vi "aptControl.vi"() -> (0 "Moving":bool, 3 "Current Position":sgl)   [LabVIEW 2012]
uses:
  <vilib>/DAQmx/write.llb/DAQmx Write (Digital 1D Bool 1Chan 1Samp).vi
  <vilib>/DAQmx/write.llb/DAQmx Write (Analog Wfm 1Chan NSamp).vi
  <vilib>/DAQmx/read.llb/DAQmx Read (Analog Wfm 1Chan NSamp).vi
  <vilib>/DAQmx/miscellaneous.llb/DAQmx Fill In Error Info.vi
  <vilib>/Analysis/baseanly.llb/Mean (DBL).vi
  <vilib>/Utility/file.llb/Write To Spreadsheet File (DBL).vi
  <vilib>/Utility/file.llb/Read From Spreadsheet File (DBL).vi
  <vilib>/gmath/NI_Gmath.lvlib
  <vilib>/Analysis/NI_AALBase.lvlib
panel:
  out "Power Min&Max":i32[](array[numeric])
  out "Setup":i32
  out "MirrorPosition":sgl
  out "SavePath":path
  out "MinPos":sgl
  out "MaxPos":sgl
  out "Scaner":string
  in  "Tab Control":enum32{"Control", "Curve", "Calibrate"}(tab)
  in  "Shutter":bool
  in  "Power (mW)":dbl format="%#.0f"
  in  "Possition (0:360)":dbl format="%#.2f"
  in  "Up":bool
  in  "Down":bool
  in  "Mirror\nOverride":bool
  in  "Galvo":bool=TRUE caption="AOD"
  in  "Lens":u16(ring)=10 items=["4X"=4, "10X"=10, "16X"=16, "20X"=20, "25X"=25, "40X"=40, "60X"=60]
  out "Error/Wait":bool
  in  "Home":bool
  in  "stop":bool
  in  "Auto":bool
  out "Calibration Used":string
  out "Curve":cluster{"all rows":dbl[], "all rows":dbl[]}(graph)
  out "Curve 2":cluster{i32[], i32[]}(graph)
  in  "Path":path=path "X:/2Pcalibration"
  in  "Start Calibration":bool
  in  "WaveLengths":dbl[](array[numeric])=[800.0, 890.0]
  out "Finished":bool
  in  "quit":bool
  out "Remaining\n min":dbl format="%#.2f"
  out "Acquiring":bool
  out "Waiting":bool
  out "Moving 2":bool
  in  "Repetitions":dbl=1.0
  in  "Step Size":dbl=4.0
  out "Current mW":dbl format="%#.0f"
  out "Old possition":sgl
  in  "AOD motor":refnum<k7>(container)
  in  "Target Position":dbl
  in  "Attenuator motor":refnum<k7>(container)
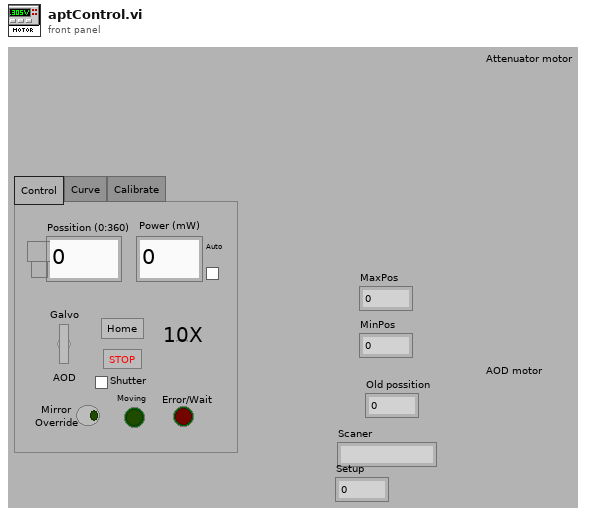
[diagram p1: front panel]
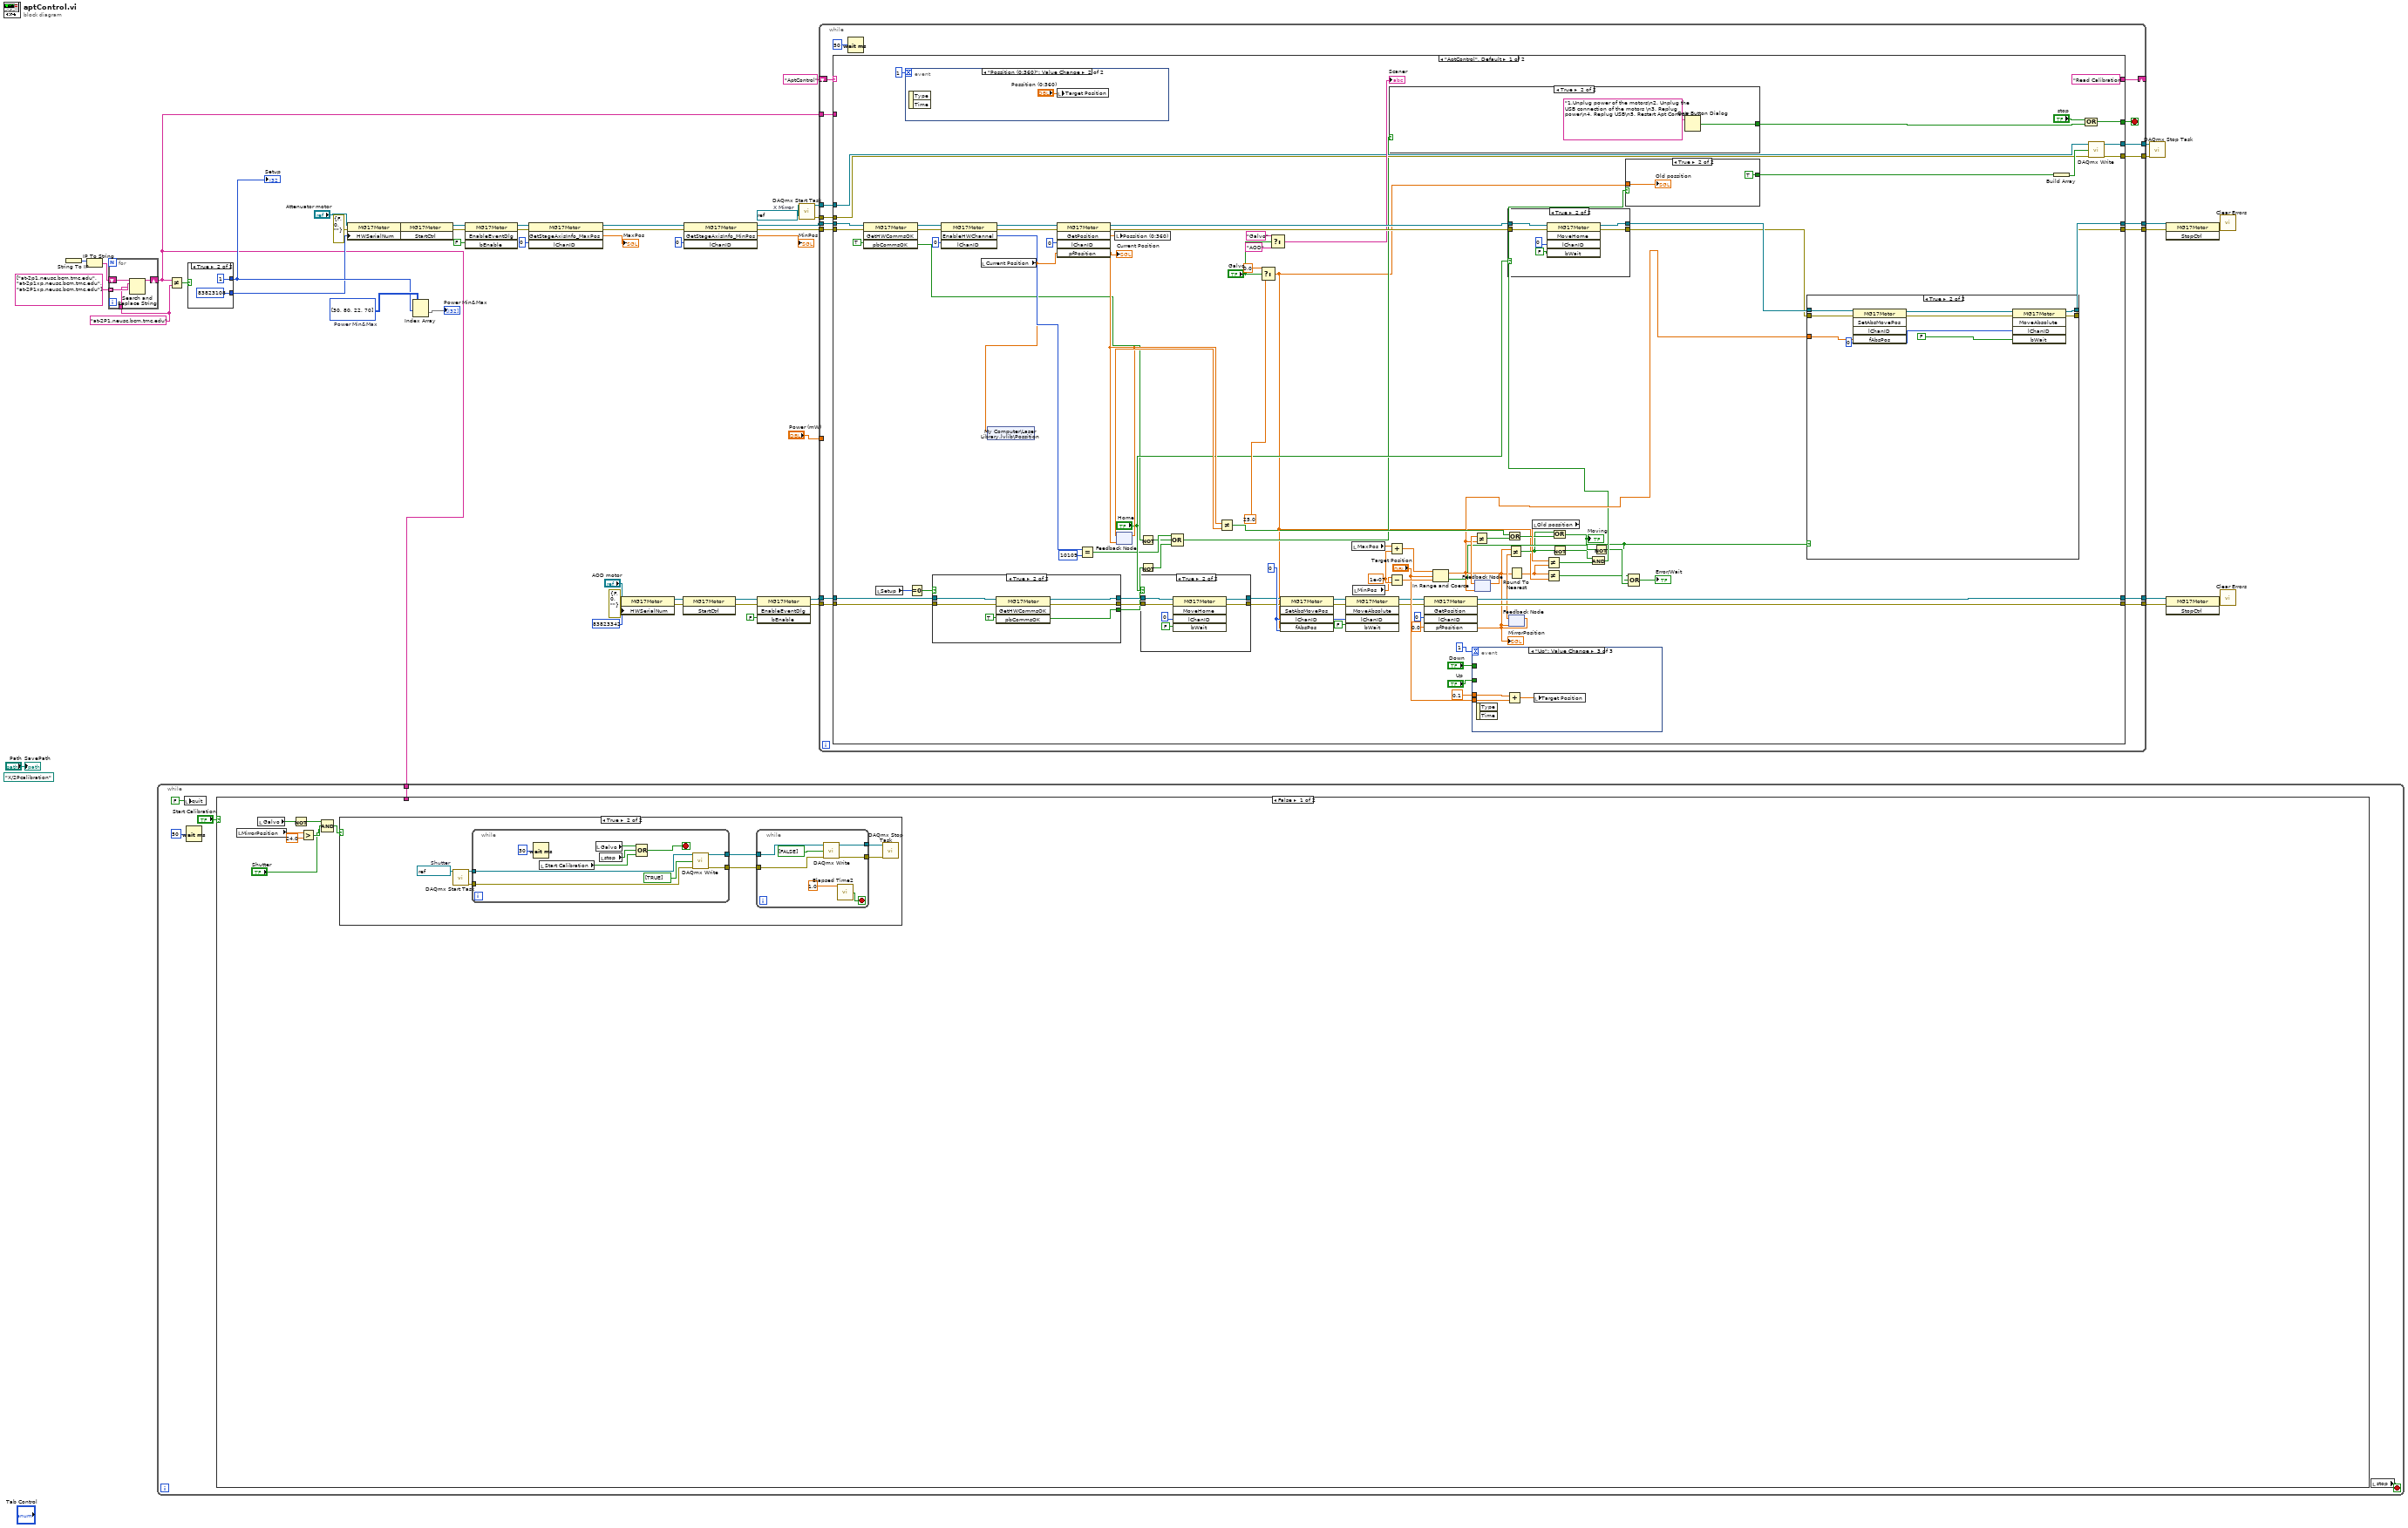
[diagram p0: block diagram]
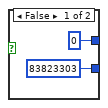
[diagram p2: hidden frame]
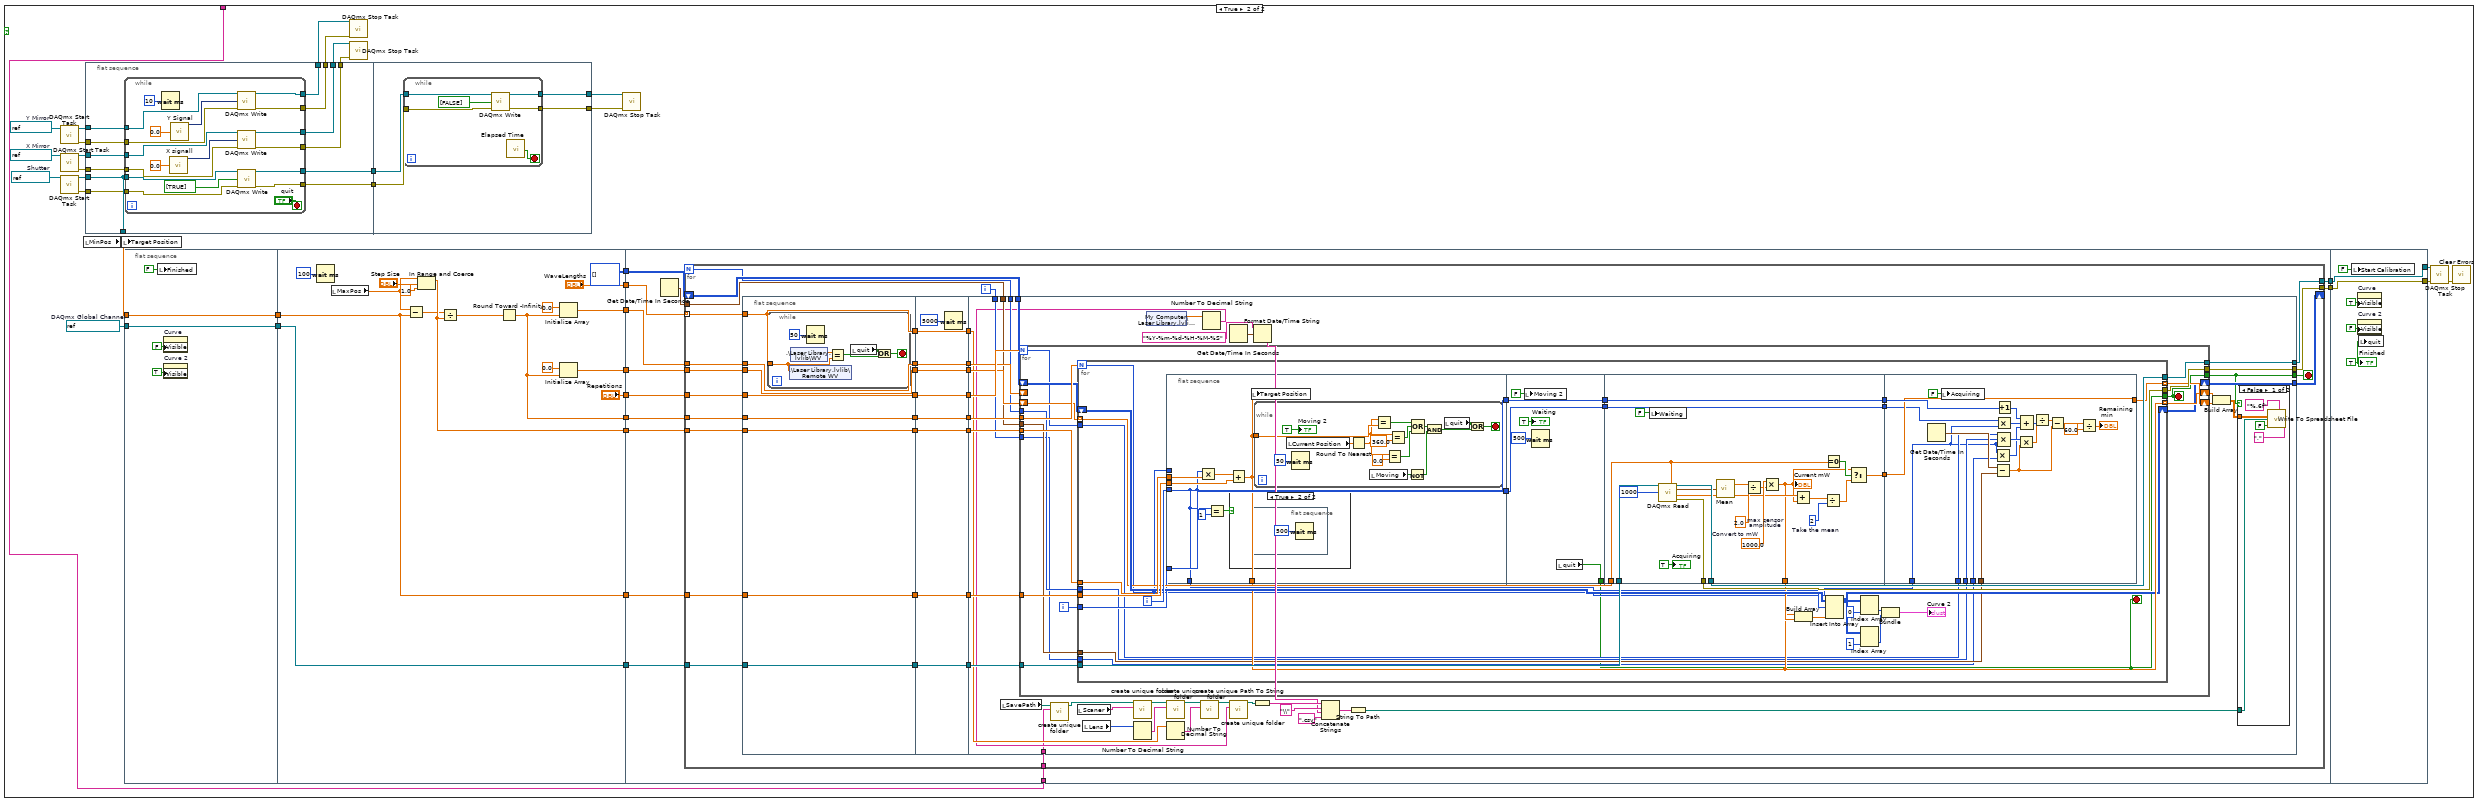
[diagram p4: hidden frame]
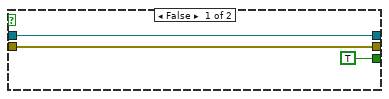
[diagram p7: hidden frame]
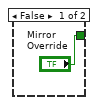
[diagram p9: hidden frame]
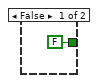
[diagram p10: hidden frame]
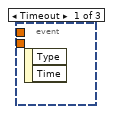
[diagram p11: hidden frame]
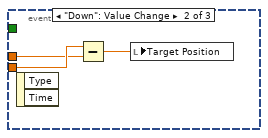
[diagram p12: hidden frame]
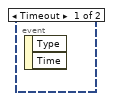
[diagram p13: hidden frame]
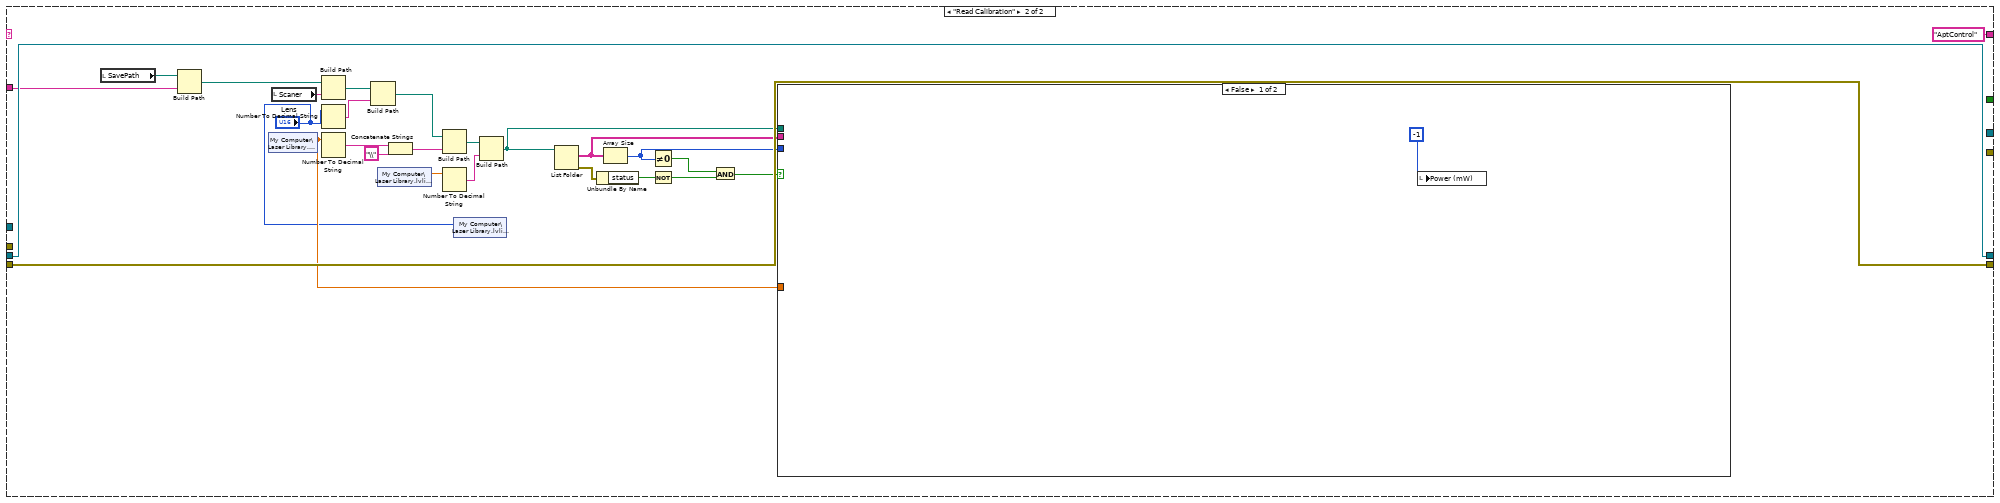
[diagram p16: hidden frame]
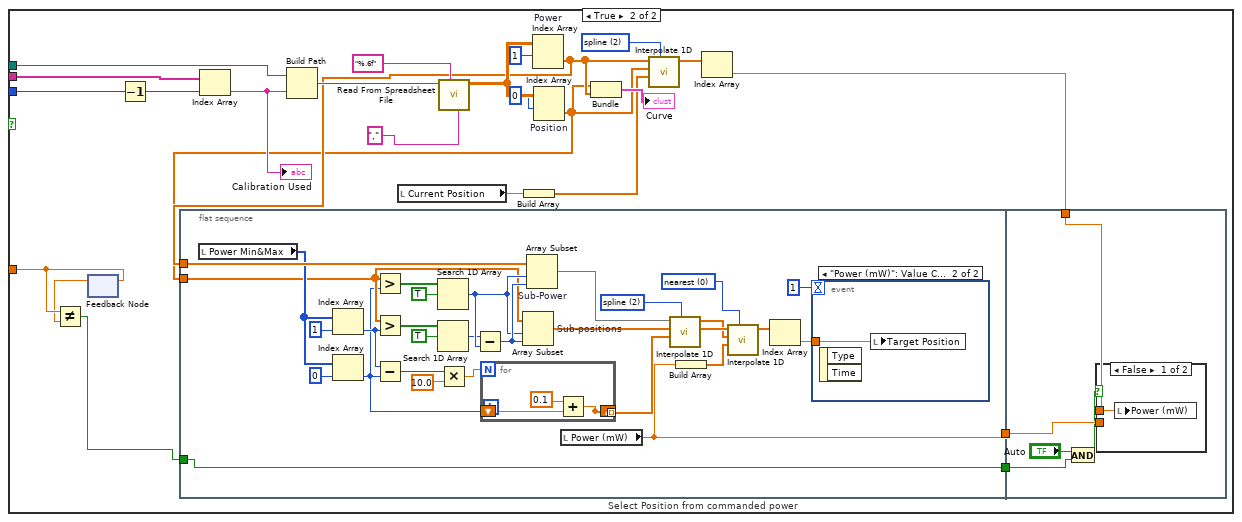
[diagram p17: hidden frame]
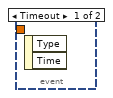
[diagram p18: hidden frame]
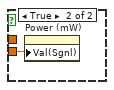
[diagram p19: hidden frame]
diagram:
  w2 = "at-2P1.neusc.bcm.tmc.edu"
  w11 = i32[][] [[30, 80], [22, 70]]  # Power Min&Max
  (unwired) path "X:/2Pcalibration"
  w20 = refnum<k21> "FlipMirror"  # X Mirror
  n1 = String To IP() -> (0:w8:u32)  [unwired: 1 in]
  n2 = IP To String(2:w8) -> (0:w3:string)  [unwired: 1 in]
  n3 = for {
    tunnel: string[] ["at-2p1.neusc.bcm.tmc.edu", "at-2p1xp.neusc.bcm.tmc.edu", "at-2P1xp.neusc.bcm.tmc.edu"] -> [w55] mode=indexing
    shift-right: [w53] -> w1
    shift-left: w3 -> [w54]
    tunnel: w2 -> [w52]
    n4 = Search and Replace String(input string=w54, search string=w55, replace string=w52) -> (result string=w53:string)  [unwired: 5 in, 3 out]
  }
  n5 = while {
    tunnel: w1 -> [w56]
    stop <- w59 stop-if-true
    n6 = local write "quit"(FALSE) -> ()
    n7 = Wait (ms)(milliseconds to wait=u32 50) -> ()  [unwired: 1 out]
    n8 = case shown="False" "Start Calibration" {
      tunnel: w56 -> [_ w92]
      frame False {
        n9 = local read "MirrorPosition"() -> (w67:sgl)
        n10 = local read "Galvo"() -> (w65:bool)
        n11 = Not(x=w65) -> (.not. x?=w66:bool)
        n12 = Greater?(x=w67, y=sgl 24.0) -> (0:w64:bool)
        n13 = Compound Arithmetic op=AND(w66, w64, "Shutter") -> (w62:bool)
        n14 = case shown="True" w62 {
          frame False {
          }
          frame True {
            w74 = refnum<k21> "Shutter"  # Shutter
            n15 = call <vilib>:"DAQmx Start Task.vi"("task/channels in"=w74) -> ("task out"=w73:refnum<k21>, "error out"=w72:errorcluster)  [unwired: 13 in]
            n16 = while {
              tunnel: w73 -> [w90]
              tunnel: w72 -> [w89]
              tunnel: [w88] -> w71
              tunnel: [w87] -> w70
              stop <- w84 stop-if-true
              n17 = Wait (ms)(milliseconds to wait=u32 30) -> ()  [unwired: 1 out]
              n18 = local read "Start Calibration"() -> (w85:bool)
              n19 = local read "Galvo"() -> (w82:bool)
              n20 = local read "stop"() -> (w86:bool)
              n21 = Compound Arithmetic op=OR(w82, w86, w85) -> (w84:bool)
              n22 = call-poly <vilib>:"DAQmx Write.vi"("task/channels in"=w90, "data"=bool[] [TRUE], "error in"=w89) -> ("task out"=w88:refnum<k21>, "error out"=w87:errorcluster)  [unwired: 10 in, 1 out]
            }
            n23 = while {
              tunnel: w71 -> [w81]
              tunnel: w70 -> [w80]
              tunnel: [w79] -> w69
              tunnel: [w78] -> w68
              stop <- w76 stop-if-true
              n24 = call-poly <vilib>:"DAQmx Write.vi"("task/channels in"=w81, "data"=bool[] [FALSE], "error in"=w80) -> ("task out"=w79:refnum<k21>, "error out"=w78:errorcluster)  [unwired: 10 in, 1 out]
              n25 = call "Elapsed Time2"("Time Target (s)"=1.0) -> ("Time has Elapsed"=w76:bool)  [unwired: 11 in, 7 out]
            }
            n26 = call <vilib>:"DAQmx Stop Task.vi"("task/channels in"=w69, "error in"=w68) -> ()  [unwired: 12 in, 2 out]
          }
        }
      }
      frame True {
        w100 = refnum<k21> "Y Mirror"  # Y Mirror
        w101 = refnum<k21> "X Mirror"  # X Mirror
        w102 = refnum<k21> "Shutter"  # Shutter
        w109 = refnum<k21> "PowerMeter"  # DAQmx Global Channel
        n27 = call <vilib>:"DAQmx Start Task.vi"("task/channels in"=w100) -> ("task out"=w99:refnum<k21>, "error out"=w94:errorcluster)  [unwired: 13 in]
        n28 = call <vilib>:"DAQmx Start Task.vi"("task/channels in"=w101) -> ("task out"=w97:refnum<k21>, "error out"=w95:errorcluster)  [unwired: 13 in]
        n29 = call <vilib>:"DAQmx Start Task.vi"("task/channels in"=w102) -> ("task out"=w98:refnum<k21>, "error out"=w96:errorcluster)  [unwired: 13 in]
        n30 = local read "MinPos"() -> (w93:sgl)
        n31 = flat-sequence {
          tunnel: [w131] -> _
          tunnel: w97 -> [w139]
          tunnel: [w138] -> w114
          tunnel: [w137] -> w113
          tunnel: [w136] -> w106
          tunnel: [w135] -> w105
          tunnel: [w134] -> w104
          tunnel: [w133] -> w103
          tunnel: w99 -> [w132]
          tunnel: w98 -> [w131]
          tunnel: w96 -> [w130]
          tunnel: w95 -> [w129]
          tunnel: w94 -> [w128]
          tunnel: w114 -> [w162]
          tunnel: [w161] -> w108
          tunnel: [w160] -> w107
          tunnel: w113 -> [w159]
          frame #0 {
            n32 = while {
              tunnel: w131 -> [w153]
              tunnel: w139 -> [w155]
              tunnel: w132 -> [w154]
              tunnel: [w151] -> w138
              tunnel: [w150] -> w137
              tunnel: [w147] -> w136
              tunnel: [w146] -> w135
              tunnel: [w145] -> w134
              tunnel: [w144] -> w133
              tunnel: w130 -> [w143]
              tunnel: w129 -> [w142]
              tunnel: w128 -> [w141]
              stop <- "quit" stop-if-true
              n33 = Wait (ms)(milliseconds to wait=u32 10) -> ()  [unwired: 1 out]
              n34 = call "X signall"("Amplitude"=0.0) -> ("Sine"=w149:dynamicdata)  [unwired: 13 in, 1 out]
              n35 = call "Y Signal"("Amplitude"=0.0) -> ("Sine"=w148:dynamicdata)  [unwired: 13 in, 1 out]
              n36 = call-poly <vilib>:"DAQmx Write.vi"("task/channels in"=w154, "data"=w148, "error in"=w141) -> ("task out"=w145:refnum<k21>, "error out"=w144:errorcluster)  [unwired: 10 in, 1 out]
              n37 = call-poly <vilib>:"DAQmx Write.vi"("task/channels in"=w155, "data"=w149, "error in"=w142) -> ("task out"=w147:refnum<k21>, "error out"=w146:errorcluster)  [unwired: 10 in, 1 out]
              n38 = call-poly <vilib>:"DAQmx Write.vi"("task/channels in"=w153, "data"=bool[] [TRUE], "error in"=w143) -> ("task out"=w151:refnum<k21>, "error out"=w150:errorcluster)  [unwired: 10 in, 1 out]
            }
          }
          frame #1 {
            n39 = while {
              tunnel: w162 -> [w167]
              tunnel: [w165] -> w161
              tunnel: [w164] -> w160
              tunnel: w159 -> [w163]
              stop <- w168 stop-if-true
              n40 = call-poly <vilib>:"DAQmx Write.vi"("task/channels in"=w167, "data"=bool[] [FALSE], "error in"=w163) -> ("task out"=w165:refnum<k21>, "error out"=w164:errorcluster)  [unwired: 10 in, 1 out]
              n41 = call "Elapsed Time"() -> ("Time has Elapsed"=w168:bool)  [unwired: 12 in, 7 out]
            }
          }
        }
        n42 = local write "Target Position"(w93) -> ()
        n43 = flat-sequence {
          tunnel: w109 -> [w172]
          tunnel: w93 -> [w173]
          tunnel: [w173] -> w127
          tunnel: [w172] -> w126
          tunnel: [w188] -> w125
          tunnel: ["Repetitions"] -> w124
          tunnel: [w187] -> w123
          tunnel: [w190] -> w122
          tunnel: [w186] -> w121
          tunnel: [w185] -> w120
          tunnel: [i32[][] []] -> w119
          tunnel: ["WaveLengths"] -> w118
          tunnel: [w184] -> w117
          tunnel: w127 -> [w188]
          tunnel: w126 -> [w190]
          tunnel: w125 -> [w203]
          tunnel: w124 -> [w202]
          tunnel: w123 -> [w201]
          tunnel: w122 -> [w200]
          tunnel: w121 -> [w198]
          tunnel: w120 -> [w197]
          tunnel: w119 -> [w195]
          tunnel: w118 -> [w196]
          tunnel: w117 -> [w199]
          tunnel: [w194] -> w116
          tunnel: [w193] -> w115
          tunnel: w92 -> [w191]
          tunnel: [w431] -> w110
          tunnel: [w432] -> w111
          tunnel: w116 -> [w432]
          tunnel: w115 -> [w431]
          frame #0 {
            n44 = local write "Finished"(FALSE ("Finished")) -> ()
            n45 = property on="Curve" class="XYGraph (strict)"("Visible"=FALSE) -> ()  [unwired: 2 in, 2 out]
            n46 = property on="Curve 2" class="XYGraph (strict)"("Visible"=TRUE) -> ()  [unwired: 2 in, 2 out]
          }
          frame #1 {
            n47 = Wait (ms)(milliseconds to wait=u32 100) -> ()  [unwired: 1 out]
            n48 = local read "MaxPos"() -> (w174:sgl)
            n49 = Subtract(x=w174, y=w188) -> (x-y=w179:sgl)
            n50 = In Range and Coerce(upper limit=w174, x="Step Size", lower limit=1.0) -> (coerced(x)=w187:dbl)  [unwired: 1 out]
            n51 = Divide(x=w179, y=w187) -> (x/y=w180:dbl)
            n52 = Round Toward -Infinity(1:w180) -> (0:w186:dbl)
            n53 = Initialize Array(0.0 ("element"), w186) -> (w185:dbl[])
            n54 = Initialize Array(0.0 ("element"), w186) -> (w184:dbl[])
          }
          frame #2 {
            n55 = Get Date/Time In Seconds() -> (seconds since 1Jan1904=w192:timestamp)
            n56 = for {
              N -> [w207]
              tunnel: w203 -> [w236]
              tunnel: w202 -> [w235]
              tunnel: w201 -> [w234]
              tunnel: w200 -> [w233]
              tunnel: [w232] -> w194
              tunnel: [w231] -> w193
              tunnel: w199 -> [w230]
              tunnel: w198 -> [w229]
              tunnel: w197 -> [w228]
              tunnel: w196 -> [w227] mode=indexing
              shift-right: [w209] -> _
              shift-left: w195 -> [w210]
              tunnel: w192 -> [w208]
              tunnel: w191 -> [w204]
              i -> [w206]
              stop <- w205 stop-if-true
              n57 = flat-sequence {
                tunnel: w227 -> [w237]
                tunnel: w228 -> [w238]
                tunnel: w229 -> [w239]
                tunnel: w230 -> [w240]
                tunnel: w233 -> [w241]
                tunnel: w234 -> [w242]
                tunnel: w235 -> [w243]
                tunnel: w236 -> [w244]
                tunnel: [w244] -> w226
                tunnel: [w243] -> w224
                tunnel: [w242] -> w222
                tunnel: [w241] -> w220
                tunnel: [w240] -> w218
                tunnel: [w239] -> w216
                tunnel: [w238] -> w214
                tunnel: [w237] -> w212
                tunnel: w226 -> [w259]
                tunnel: [w259] -> w225
                tunnel: w224 -> [w258]
                tunnel: [w258] -> w223
                tunnel: w222 -> [w257]
                tunnel: [w257] -> w221
                tunnel: w220 -> [w256]
                tunnel: [w256] -> w219
                tunnel: w218 -> [w255]
                tunnel: [w255] -> w217
                tunnel: w216 -> [w254]
                tunnel: [w254] -> w215
                tunnel: w214 -> [w253]
                tunnel: [w253] -> w213
                tunnel: w212 -> [w252]
                tunnel: [w252] -> w211
                tunnel: [w297] -> w209
                tunnel: [w298] -> w231
                tunnel: [w299] -> w232
                tunnel: w206 -> [w271]
                tunnel: w207 -> [w272]
                tunnel: w208 -> [w273]
                tunnel: w210 -> [w274]
                tunnel: w211 -> [w275]
                tunnel: w213 -> [w290]
                tunnel: w215 -> [w291]
                tunnel: w217 -> [w292]
                tunnel: w219 -> [w293]
                tunnel: w221 -> [w294]
                tunnel: w223 -> [w295]
                tunnel: w225 -> [w296]
                tunnel: [w262] -> w205
                tunnel: w204 -> [w260]
                frame #0 {
                  n58 = while {
                    tunnel: w237 -> [w249]
                    stop <- w245 stop-if-true
                    n59 = shared-variable ".\\Laser Library.lvlib\\Remote WV"(w249) -> ()  [unwired: 1 in, 1 out]
                    n60 = shared-variable ".\\Laser Library.lvlib\\WV"() -> (w248:dbl)  [unwired: 1 in, 1 out]
                    n61 = Wait (ms)(milliseconds to wait=u32 50) -> ()  [unwired: 1 out]
                    n62 = Equal?(x=w248, y=w249) -> (x = y?=w246:bool)
                    n63 = local read "quit"() -> (w247:bool)
                    n64 = Or(x=w247, y=w246) -> (x .or. y?=w245:bool)
                  }
                }
                frame #1 {
                  n65 = Wait (ms)(milliseconds to wait=u32 5000) -> ()  [unwired: 1 out]
                }
                frame #2 {
                  n66 = local read "SavePath"() -> (w261:path)
                  n67 = for {
                    N: w295 -> [w307]
                    tunnel: w291 -> [w321]
                    tunnel: w296 -> [w320]
                    tunnel: w294 -> [w319]
                    tunnel: w293 -> [w318]
                    tunnel: [w317] -> w299
                    tunnel: [w316] -> w298
                    shift-right: [w315] -> w277
                    shift-left: w292 -> [w313]
                    shift-right: [w314] -> w278
                    shift-left: w290 -> [_]
                    shift-right: [w312] -> w297
                    shift-left: w274 -> [w311]
                    tunnel: w273 -> [w309]
                    tunnel: w272 -> [w308]
                    tunnel: w271 -> [w306]
                    tunnel: [w305] -> w262
                    i -> [w310]
                    stop <- w305 stop-if-true
                    n68 = for {
                      N: w321 -> [w325]
                      tunnel: w320 -> [w354]
                      tunnel: w319 -> [w353]
                      tunnel: w318 -> [w351]
                      tunnel: [w350] -> w317
                      tunnel: [w349] -> w316
                      tunnel: [w324] -> w315 mode=indexing
                      tunnel: w313 -> [w346] mode=indexing
                      tunnel: [w342] -> w314 mode=indexing
                      shift-right: [w339] -> w312
                      shift-left: w311 -> [w347]
                      tunnel: w310 -> [w336]
                      tunnel: w309 -> [w335]
                      tunnel: w308 -> [w334]
                      tunnel: w307 -> [w333]
                      tunnel: w306 -> [w332]
                      tunnel: [w323] -> w305
                      i -> [w352]
                      stop <- w323 stop-if-true
                      n69 = flat-sequence {
                        tunnel: w352 -> [w358]
                        tunnel: w353 -> [w362]
                        tunnel: w354 -> [w359]
                        tunnel: [w355] -> w342
                        tunnel: [w358] -> w343
                        tunnel: w336 -> [w361]
                        tunnel: [w361] -> w329
                        tunnel: [w358] -> w326
                        tunnel: w325 -> [_]
                        tunnel: [w384] -> w330
                        tunnel: w329 -> [w384]
                        tunnel: [w383] -> w327
                        tunnel: w326 -> [w383]
                        tunnel: [w380] -> w323
                        tunnel: w351 -> [w405]
                        tunnel: [w404] -> w350
                        tunnel: [w403] -> w349
                        tunnel: w346 -> [w389]
                        tunnel: [w397] -> w348
                        tunnel: [w386] -> w345
                        tunnel: [w391] -> w331
                        tunnel: w330 -> [w391]
                        tunnel: [w390] -> w328
                        tunnel: w327 -> [w390]
                        tunnel: w348 -> [w420]
                        tunnel: w335 -> [w425]
                        tunnel: w334 -> [w424]
                        tunnel: w333 -> [w423]
                        tunnel: w325 -> [w412]
                        tunnel: w332 -> [w413]
                        tunnel: w331 -> [w414]
                        tunnel: w328 -> [w422]
                        tunnel: [w420] -> w324
                        frame #0 {
                          n70 = Multiply(x=w358, y=w362) -> (x*y=w360:dbl)
                          n71 = Equal?(x=w358, y=1) -> (x = y?=w357:bool)
                          n72 = Add(x=w360, y=w359) -> (x+y=w355:dbl)
                          n73 = case shown="True" w357 {
                            frame False {
                            }
                            frame True {
                              n74 = flat-sequence {
                                frame #0 {
                                n75 = Wait (ms)(milliseconds to wait=u32 500) -> ()  [unwired: 1 out]
                                }
                              }
                            }
                          }
                          n76 = local write "Target Position"(w355) -> ()
                          n77 = while {
                            tunnel: w355 -> [w378]
                            stop <- w365 stop-if-true
                            n78 = local read "Current Position"() -> (w367:sgl)
                            n79 = Wait (ms)(milliseconds to wait=u32 50) -> ()  [unwired: 1 out]
                            n80 = Round To Nearest(number=w367) -> (nearest integer value=w372:sgl)
                            n81 = local read "Moving"() -> (w368:bool)
                            n82 = Equal?(x=w372, y=w378) -> (x = y?=w376:bool)
                            n83 = Equal?(x=w372, y=0.0) -> (x = y?=w373:bool)
                            n84 = Equal?(x=w372, y=360.0) -> (x = y?=w374:bool)
                            n85 = Not(x=w368) -> (.not. x?=w377:bool)
                            n86 = Compound Arithmetic op=OR(w376, w374, w373) -> (w375:bool)
                            n87 = And(x=w375, y=w377) -> (x .and. y?=w366:bool)
                            n88 = local read "quit"() -> (w364:bool)
                            n89 = Or(x=w364, y=w366) -> (x .or. y?=w365:bool)
                            "Moving 2" <- TRUE
                          }
                        }
                        frame #1 {
                          n90 = local write "Moving 2"(FALSE) -> ()
                          n91 = Wait (ms)(milliseconds to wait=u32 500) -> ()  [unwired: 1 out]
                          n92 = local read "quit"() -> (w380:bool)
                          "Waiting" <- TRUE
                        }
                        frame #2 {
                          w392 = 2.0  # max sensor  amplitude
                          w394 = 1000.0  # Convert to mW
                          w400 = 2  # Take the mean
                          n93 = local write "Waiting"(FALSE) -> ()
                          n94 = call-poly <vilib>:"DAQmx Read.vi"("task/channels in"=w405, "number of samples per channel"=1000) -> ("task out"=w404:refnum<k21>, "data"=w395:waveform(dbl), "error out"=w403:errorcluster)  [unwired: 1 in, 10 out]
                          n95 = call-poly <vilib>:"Mean.vi"("X"=w395) -> ("mean"=w396:dbl)  [unwired: 1 out]
                          n96 = Divide(x=w396, y=w392) -> (x/y=w393:dbl)
                          n97 = Multiply(x=w394, y=w393) -> (x*y=w386:dbl)
                          "Current mW" <- w386
                          n98 = Add(x=w389, y=w386) -> (x+y=w399:dbl)
                          n99 = Divide(x=w399, y=w400) -> (x/y=w398:dbl)
                          n100 = Equal To 0?(x=w389) -> (x = 0?=w401:bool)
                          n101 = Select(t=w386, s=w401, f=w398) -> (s? t:f=w397:dbl)
                          "Acquiring" <- TRUE ("Acquiring")
                        }
                        frame #3 {
                          n102 = Get Date/Time In Seconds() -> (seconds since 1Jan1904=w426:timestamp)
                          n103 = local write "Acquiring"(FALSE ("Acquiring")) -> ()
                          n104 = Multiply(x=w412, y=w413) -> (x*y=w409:i32)
                          n105 = Subtract(x=w426, y=w425) -> (x-y=w417:dbl)
                          n106 = Multiply(x=w414, y=w412) -> (x*y=w410:i32)
                          n107 = Increment(x=w422) -> (x+1=w411:i32)
                          n108 = Compound Arithmetic op=MULTIPLY(w423, w424, w412) -> (w419:i32)
                          n109 = Multiply(x=w419, y=w417) -> (x*y=w418:dbl)
                          n110 = Compound Arithmetic op=ADD(w411, w410, w409) -> (w408:i32)
                          n111 = Divide(x=w418, y=w408) -> (x/y=w416:dbl)
                          n112 = Subtract(x=w416, y=w417) -> (x-y=w415:dbl)
                          n113 = Divide(x=w415, y=60.0) -> (x/y=→"Remaining\n min":dbl)
                        }
                      }
                      n114 = Build Array(w342, w345) -> (w344:dbl[])
                      n115 = Insert Into Array(array=w347, index (row)=w343, new element=w344) -> (w339:i32[][])  [unwired: 1 in]
                      n116 = Index Array(array=w339, index (col)=0 ("index")) -> (element=w340:i32[])  [unwired: 1 in]
                      n117 = Index Array(array=w339, index (col)=1 ("index")) -> (element=w337:i32[])  [unwired: 1 in]
                      n118 = Bundle(w340, w337) -> (→"Curve 2":cluster{i32[], i32[]})  [unwired: 1 in]
                    }
                  }
                  n119 = call "create unique folder.vi"("string"=w260, "path 2"=w261) -> ("path"=w270:path)  [unwired: 9 in]
                  n120 = local read "Scaner"() -> (w263:string)
                  n121 = local read "Lens"() -> (w264:u16)
                  n122 = call "create unique folder.vi"("string"=w263, "path 2"=w270) -> ("path"=w269:path)  [unwired: 9 in]
                  n123 = Number To Decimal String(number=w264) -> (decimal integer string=w279:string)  [unwired: 1 in]
                  n124 = shared-variable "My Computer\\Laser Library.lvlib\\GDD"() -> (w268:dbl)  [unwired: 1 in, 1 out]
                  n125 = call "create unique folder.vi"("string"=w279, "path 2"=w269) -> ("path"=w280:path)  [unwired: 9 in]
                  n126 = Number To Decimal String(number=w275) -> (decimal integer string=w287:string)  [unwired: 1 in]
                  n127 = call "create unique folder.vi"("string"=w287, "path 2"=w280) -> ("path"=w267:path)  [unwired: 9 in]
                  n128 = Number To Decimal String(number=w268) -> (decimal integer string=w265:string)  [unwired: 1 in]
                  n129 = Get Date/Time In Seconds() -> (seconds since 1Jan1904=w289:timestamp)
                  n130 = call "create unique folder.vi"("string"=w265, "path 2"=w267) -> ("path"=w266:path)  [unwired: 9 in]
                  n131 = Path To String(path=w266) -> (string=w286:string)
                  n132 = Format Date/Time String(time format string (%c)="%Y-%m-%d-%H-%M-%S", seconds (now)=w289) -> (date/time string=w284:string)  [unwired: 1 in]
                  n133 = Concatenate Strings(w286, "\\" ("string"), w284, ".csv" ("string")) -> (w283:string)
                  n134 = String To Path(string=w283) -> (path=w282:path)
                  n135 = Build Array(w278, w277) -> (w276:dbl[][])
                  n136 = case shown="False" w262 {
                    tunnel: w282 -> [w301 _]
                    tunnel: w276 -> [w300 _]
                    frame False {
                      n137 = call-poly <vilib>:"Write To Spreadsheet File.vi"("delimiter (\\t)"="," ("delimiter (\\t)"), "format (%.3f)"="%.6f", "append to file? (new file:F)"=FALSE, "2D data"=w300, "file path (dialog if empty)"=w301) -> ()  [unwired: 2 in, 2 out]
                    }
                    frame True {
                    }
                  }
                }
              }
            }
          }
          frame #3 {
            w430 = TRUE ("Finished")
            n138 = local write "Start Calibration"(FALSE) -> ()
            n139 = property on="Curve" class="XYGraph (strict)"("Visible"=TRUE) -> ()  [unwired: 2 in, 2 out]
            n140 = property on="Curve 2" class="XYGraph (strict)"("Visible"=FALSE) -> ()  [unwired: 2 in, 2 out]
            n141 = local write "quit"(w430) -> ()
            "Finished" <- w430
          }
        }
        n142 = call <vilib>:"DAQmx Stop Task.vi"("task/channels in"=w104, "error in"=w103) -> ()  [unwired: 12 in, 2 out]
        n143 = call <vilib>:"DAQmx Stop Task.vi"("task/channels in"=w106, "error in"=w105) -> ()  [unwired: 12 in, 2 out]
        n144 = call <vilib>:"DAQmx Stop Task.vi"("task/channels in"=w108, "error in"=w107) -> ()  [unwired: 12 in, 2 out]
        n145 = call <vilib>:"DAQmx Stop Task.vi"("task/channels in"=w111, "error in"=w110) -> ("error out"=w112:errorcluster)  [unwired: 13 out]
        n146 = call <vilib>:"Clear Errors.vi"("error in (no error)"=w112) -> ()  [unwired: 6 in, 1 out]
      }
    }
    n147 = local read "stop"() -> (w59:bool)
  }
  n148 = Not Equal?(x=w1, y=w2) -> (x != y?=w7:bool)
  n149 = case shown="True" w7 {
    tunnel: [0 1] -> w6
    tunnel: [83823303 83823108] -> w5
    frame False {
    }
    frame True {
    }
  }
  "Setup" <- w6
  n150 = property class="MG17Motor"(reference="Attenuator motor", error in=errorcluster {"status"=FALSE, "code"=0, "source"=""} ("error in (no error)"), "HWSerialNum"=w5) -> (reference out=w50:refnum<k7>, error out=w49:errorcluster)
  n151 = invoke class="MG17Motor" method="StartCtrl"(reference=w50, error in=w49) -> (reference out=w38:refnum<k7>, error out=w37:errorcluster)  [unwired: 1 in, 1 out]
  n152 = Index Array(array=w11, index (row)=w6) -> (element=→"Power Min&Max":i32[])  [unwired: 1 in]
  n153 = invoke class="MG17Motor" method="EnableEventDlg"(reference=w38, error in=w37, "bEnable"=FALSE) -> (reference out=w36:refnum<k7>, error out=w35:errorcluster)  [unwired: 1 in, 2 out]
  n154 = invoke class="MG17Motor" method="GetStageAxisInfo_MaxPos"(reference=w36, error in=w35, "lChanID"=0) -> (reference out=w41:refnum<k7>, error out=w40:errorcluster, "GetStageAxisInfo_MaxPos"=→"MaxPos":sgl)  [unwired: 1 in, 1 out]
  n155 = property class="MG17Motor"(reference="AOD motor", error in=errorcluster {"status"=FALSE, "code"=0, "source"=""} ("error in (no error)"), "HWSerialNum"=83823342) -> (reference out=w30:refnum<k7>, error out=w31:errorcluster)
  n156 = invoke class="MG17Motor" method="StartCtrl"(reference=w30, error in=w31) -> (reference out=w33:refnum<k7>, error out=w34:errorcluster)  [unwired: 1 in, 1 out]
  n157 = invoke class="MG17Motor" method="GetStageAxisInfo_MinPos"(reference=w41, error in=w40, "lChanID"=0) -> (reference out=w48:refnum<k7>, error out=w43:errorcluster, "GetStageAxisInfo_MinPos"=→"MinPos":sgl)  [unwired: 1 in, 1 out]
  n158 = invoke class="MG17Motor" method="EnableEventDlg"(reference=w33, error in=w34, "bEnable"=FALSE) -> (reference out=w28:refnum<k7>, error out=w23:errorcluster)  [unwired: 1 in, 2 out]
  n159 = call <vilib>:"DAQmx Start Task.vi"("task/channels in"=w20) -> ("task out"=w17:refnum<k21>, "error out"=w16:errorcluster)  [unwired: 13 in]
  n160 = while {
    tunnel: w48 -> [w453]
    tunnel: [w450] -> w46
    tunnel: [w451] -> w45
    tunnel: w43 -> [w449]
    shift-right: [w446] -> _
    shift-left: "AptControl" -> [w447]
    tunnel: w1 -> [w445]
    tunnel: w28 -> [w444]
    tunnel: [w443] -> w25
    tunnel: [w442] -> w24
    tunnel: w23 -> [w441]
    tunnel: [w440] -> w19
    tunnel: [w439] -> w18
    tunnel: w17 -> [w438]
    tunnel: w16 -> [w437]
    tunnel: "Power (mW)" -> [_]
    stop <- w448 stop-if-true
    n161 = case shown="\"AptControl\", Default" w447 {
      tunnel: w453 -> [w479 w618]
      tunnel: [w534 w618] -> w451
      tunnel: [w533 w617] -> w450
      tunnel: w449 -> [w477 w617]
      tunnel: [w527 _] -> w448
      tunnel: ["Read Calibration" "AptControl"] -> w446
      tunnel: w445 -> [_ w614]
      tunnel: w444 -> [w475 _]
      tunnel: [w505 _] -> w443
      tunnel: [w504 _] -> w442
      tunnel: w441 -> [w473 _]
      tunnel: [w486 _] -> w440
      tunnel: [w485 _] -> w439
      tunnel: w438 -> [w484 _]
      tunnel: w437 -> [w483 _]
      frame "AptControl", Default {
        w513 = 0 ("lChanID")
        w536 = 1e-07
        n162 = invoke class="MG17Motor" method="GetHWCommsOK"(reference=w479, error in=w477, "pbCommsOK"=TRUE) -> (reference out=w478:refnum<k7>, error out=w476:errorcluster, "pbCommsOK"=w467:bool)  [unwired: 1 in, 1 out]
        n163 = local read "Setup"() -> (w456:i32)
        n164 = event shown="[1] \"Possition (0:360)\": Value Change" {
          selector: _ -> [_ _]
          dyn-events: _ -> [_ _]
          timeout: 1 -> [_ _]
          event Timeout {
            n165 = event-data() -> ()  [unwired: 1 in, 2 out]
          }
          event "Possition (0:360)": Value Change {
            n166 = event-data() -> ()  [unwired: 1 in, 2 out]
            n167 = local write "Target Position"("Possition (0:360)") -> ()
          }
        }
        n168 = Equal To 0?(x=w456) -> (x = 0?=w455:bool)
        n169 = case shown="True" w455 {
          tunnel: w475 -> [w547 w552]
          tunnel: [w547 w551] -> w474
          tunnel: w473 -> [w546 w550]
          tunnel: [w546 w549] -> w472
          tunnel: [TRUE ("pbCommsOK") w548] -> w465
          frame False {
          }
          frame True {
            n170 = invoke class="MG17Motor" method="GetHWCommsOK"(reference=w552, error in=w550, "pbCommsOK"=TRUE) -> (reference out=w551:refnum<k7>, error out=w549:errorcluster, "pbCommsOK"=w548:bool)  [unwired: 1 in, 1 out]
          }
        }
        n171 = invoke class="MG17Motor" method="EnableHWChannel"(reference=w478, error in=w476, "lChanID"=0) -> (reference out=w517:refnum<k7>, error out=w516:errorcluster, "EnableHWChannel"=w515:i32)  [unwired: 1 in, 1 out]
        n172 = local read "Current Position"() -> (w454:sgl)
        n173 = shared-variable "My Computer\\Laser Library.lvlib\\Possition"(w454) -> ()  [unwired: 1 in, 1 out]
        n174 = invoke class="MG17Motor" method="GetPosition"(reference=w517, error in=w516, "lChanID"=0, "pfPosition"=w454) -> (reference out=w532:refnum<k7>, error out=w519:errorcluster, "pfPosition"=w526:sgl)  [unwired: 1 in, 2 out]
        "Current Position" <- w526
        n175 = Equal?(x=w515, y=10109) -> (x = y?=w471:bool)
        n176 = local write "Possition (0:360)"(w526) -> ()
        n177 = feedback #1(w526) -> (w541:sgl)
        n178 = feedback-in #1(w526) -> ()
        n179 = Not(x=w467) -> (.not. x?=w466:bool)
        n180 = Not(x=w465) -> (.not. x?=w464:bool)
        n181 = case shown="True" "Home" {
          tunnel: [w554 w559] -> w492
          tunnel: [w555 w558] -> w491
          tunnel: w474 -> [w554 w557]
          tunnel: w472 -> [w555 w556]
          frame False {
          }
          frame True {
            n182 = invoke class="MG17Motor" method="MoveHome"(reference=w557, error in=w556, "lChanID"=0, "bWait"=FALSE) -> (reference out=w559:refnum<k7>, error out=w558:errorcluster)  [unwired: 1 in, 3 out]
          }
        }
        n183 = Compound Arithmetic op=OR(w471, w466, w464) -> (w470:bool)
        n184 = Not Equal?(x=w526, y=w541) -> (x != y?=w540:bool)
        n185 = Select(t=sgl 0.0 ("pfPosition"), s="Galvo", f=sgl 25.0 ("pfPosition")) -> (s? t:f=w461:sgl)
        n186 = Select(t="Galvo", s="Galvo", f="AOD") -> (s? t:f=→"Scaner":string)
        n187 = invoke class="MG17Motor" method="SetAbsMovePos"(reference=w492, error in=w491, "lChanID"=w513, "fAbsPos"=w461) -> (reference out=w511:refnum<k7>, error out=w514:errorcluster)  [unwired: 1 in, 3 out]
        n188 = invoke class="MG17Motor" method="MoveAbsolute"(reference=w511, error in=w514, "lChanID"=w513, "bWait"=FALSE) -> (reference out=w507:refnum<k7>, error out=w506:errorcluster)  [unwired: 1 in, 3 out]
        n189 = local read "MaxPos"() -> (w469:sgl)
        n190 = local read "MinPos"() -> (w468:sgl)
        n191 = case shown="True" w470 {
          tunnel: [FALSE ("true") w566] -> w457
          frame False {
          }
          frame True {
            n192 = One Button Dialog(message="1.Unplug power of the motors\n2. Unplug the USB connection of the motors \n3. Replug power\n4. Replug USB\n5. Restart Apt Control") -> (true=w566:bool)  [unwired: 1 in]
          }
        }
        n193 = Add(x=w469, y=w536) -> (x+y=w537:dbl)
        n194 = Subtract(x=w468, y=w536) -> (x-y=w535:dbl)
        n195 = invoke class="MG17Motor" method="GetPosition"(reference=w507, error in=w506, "lChanID"=0, "pfPosition"=sgl 0.0) -> (reference out=w505:refnum<k7>, error out=w504:errorcluster, "pfPosition"=w499:sgl)  [unwired: 1 in, 2 out]
        "MirrorPosition" <- w499
        n196 = In Range and Coerce(upper limit=w537, x="Target Position", lower limit=w535) -> (coerced(x)=w539:dbl, In Range?=w538:bool)
        n197 = event shown="[2] \"Up\": Value Change" {
          selector: _ -> [_ _ _]
          dyn-events: _ -> [_ _ _]
          timeout: 1 -> [_ _ _]
          tunnel: "Up" -> [_ _ _]
          tunnel: "Down" -> [_ _ _]
          tunnel: 0.1 -> [_ w569 w573]
          tunnel: "Target Position" -> [_ w570 w572]
          event Timeout {
            n198 = event-data() -> ()  [unwired: 1 in, 2 out]
          }
          event "Down": Value Change {
            n199 = event-data() -> ()  [unwired: 1 in, 2 out]
            n200 = Subtract(x=w570, y=w569) -> (x-y=w568:dbl)
            n201 = local write "Target Position"(w568) -> ()
          }
          event "Up": Value Change {
            n202 = event-data() -> ()  [unwired: 1 in, 2 out]
            n203 = Add(x=w573, y=w572) -> (x+y=w571:dbl)
            n204 = local write "Target Position"(w571) -> ()
          }
        }
        n205 = feedback #2(w539) -> (w543:dbl)
        n206 = Not Equal?(x=w543, y=w539) -> (x != y?=w542:bool)
        n207 = feedback-in #2(w539) -> ()
        n208 = Or(x=w540, y=w542) -> (x .or. y?=w482:bool)
        n209 = case shown="True" "Home" {
          tunnel: w532 -> [w576 w582]
          tunnel: w519 -> [w575 w579]
          tunnel: [w576 w578] -> w531
          tunnel: [w575 w577] -> w530
          frame False {
          }
          frame True {
            n210 = invoke class="MG17Motor" method="MoveHome"(reference=w582, error in=w579, "lChanID"=0, "bWait"=FALSE) -> (reference out=w578:refnum<k7>, error out=w577:errorcluster)  [unwired: 1 in, 3 out]
          }
        }
        n211 = feedback #3(w499) -> (w503:sgl)
        n212 = Not Equal?(x=w499, y=w503) -> (x != y?=w481:bool)
        n213 = feedback-in #3(w499) -> ()
        n214 = Round To Nearest(number=w499) -> (nearest integer value=w460:sgl)
        n215 = local read "Old possition"() -> (w500:sgl)
        n216 = Not Equal?(x=w500, y=w460) -> (x != y?=w498:bool)
        n217 = Not Equal?(x=w460, y=w461) -> (x != y?=w459:bool)
        n218 = Or(x=w481, y=w482) -> (x .or. y?=w462:bool)
        "Moving" <- w462
        n219 = Not(x=w481) -> (.not. x?=w502:bool)
        n220 = And(x=w502, y=w498) -> (x .and. y?=w501:bool)
        n221 = Not(x=w538) -> (.not. x?=w463:bool)
        n222 = case shown="True" w501 {
          tunnel: w461 -> [_ w564]
          tunnel: ["Mirror\nOverride" TRUE] -> w497
          frame False {
          }
          frame True {
            "Old possition" <- w564
          }
        }
        n223 = Compound Arithmetic op=OR(w459, w462, w463) -> (→"Error/Wait":bool)
        n224 = case shown="True" w462 {
          tunnel: w531 -> [w583 w593]
          tunnel: w539 -> [_ w589]
          tunnel: w530 -> [w584 w588]
          tunnel: [w584 w586] -> w533
          tunnel: [w583 w585] -> w534
          frame False {
          }
          frame True {
            w590 = 0 ("lChanID")
            n225 = invoke class="MG17Motor" method="SetAbsMovePos"(reference=w593, error in=w588, "lChanID"=w590, "fAbsPos"=w589) -> (reference out=w592:refnum<k7>, error out=w587:errorcluster)  [unwired: 1 in, 3 out]
            n226 = invoke class="MG17Motor" method="MoveAbsolute"(reference=w592, error in=w587, "lChanID"=w590, "bWait"=FALSE) -> (reference out=w585:refnum<k7>, error out=w586:errorcluster)  [unwired: 1 in, 3 out]
          }
        }
        n227 = Build Array(w497) -> (w487:bool[])
        n228 = Compound Arithmetic op=OR("stop", w457) -> (w527:bool)
        n229 = call-poly <vilib>:"DAQmx Write.vi"("task/channels in"=w484, "data"=w487, "error in"=w483) -> ("task out"=w486:refnum<k21>, "error out"=w485:errorcluster)  [unwired: 10 in, 1 out]
      }
      frame "Read Calibration" {
        n230 = local read "SavePath"() -> (w596:path)
        n231 = Build Path(base path=w596, name or relative path=w614) -> (appended path=w603:path)
        n232 = shared-variable "My Computer\\Laser Library.lvlib\\WV"() -> (w595:dbl)  [unwired: 1 in, 1 out]
        n233 = local read "Scaner"() -> (w597:string)
        n234 = Build Path(base path=w603, name or relative path=w597) -> (appended path=w604:path)
        n235 = Number To Decimal String(number="Lens") -> (decimal integer string=w616:string)  [unwired: 1 in]
        n236 = Number To Decimal String(number=w595) -> (decimal integer string=w605:string)  [unwired: 1 in]
        n237 = Build Path(base path=w604, name or relative path=w616) -> (appended path=w600:path)
        n238 = shared-variable "My Computer\\Laser Library.lvlib\\GDD"() -> (w602:dbl)  [unwired: 1 in, 1 out]
        n239 = Concatenate Strings(w605, "\\" ("string")) -> (w611:string)
        n240 = Build Path(base path=w600, name or relative path=w611) -> (appended path=w599:path)
        n241 = Number To Decimal String(number=w602) -> (decimal integer string=w601:string)  [unwired: 1 in]
        n242 = shared-variable "My Computer\\Laser Library.lvlib\\Lens"("Lens") -> ()  [unwired: 1 in, 1 out]
        n243 = Build Path(base path=w599, name or relative path=w601) -> (appended path=w598:path)
        n244 = List Folder(path=w598) -> (filenames=w615:string[], error out=w610:errorcluster)  [unwired: 3 in, 2 out]
        n245 = Unbundle By Name(w610) -> ("status"=w607:bool)
        n246 = Array Size(array=w615) -> (size(s)=w613:i32)
        n247 = Not Equal To 0?(x=w613) -> (x != 0?=w608:bool)
        n248 = Not(x=w607) -> (.not. x?=w606:bool)
        n249 = And(x=w608, y=w606) -> (x .and. y?=w609:bool)
        n250 = case shown="False" w609 {
          tunnel: w615 -> [_ w644]
          tunnel: w613 -> [_ w643]
          tunnel: w598 -> [_ w641]
          tunnel: w595 -> [_ w626]
          frame False {
            n251 = local write "Power (mW)"(-1) -> ()
          }
          frame True {
            w632 = 2 items=["nearest", "linear", "spline", "cubic Hermite", "Lagrange"] ("method")
            n252 = feedback-in #4(w626) -> ()
            n253 = feedback #4() -> (w625:dbl)  [unwired: 1 in]
            n254 = Not Equal?(x=w626, y=w625) -> (x != y?=w622:bool)
            n255 = Decrement(x=w643) -> (x-1=w642:i32)
            n256 = flat-sequence "Select Position from commanded power" {
              tunnel: w628 -> [w672]
              tunnel: w627 -> [w661]
              tunnel: [w657] -> w624
              tunnel: w622 -> [w645]
              tunnel: [w645] -> w621
              tunnel: w624 -> [w683]
              tunnel: w623 -> [w680]
              tunnel: w621 -> [w679]
              frame #0 {
                w656 = 2 items=["nearest", "linear", "spline", "cubic Hermite", "Lagrange"] ("method")
                w668 = 0 items=["nearest", "linear", "spline", "cubic Hermite", "Lagrange"] ("method")
                n257 = local read "Power Min&Max"() -> (w667:i32[])
                n258 = Index Array(array=w667, index=1) -> (element=w648:i32)
                n259 = Index Array(array=w667, index=0) -> (element=w647:i32)
                n260 = Greater?(x=w661, y=w647) -> (0:w666:bool[])
                n261 = Greater?(x=w661, y=w648) -> (0:w663:bool[])
                n262 = Subtract(x=w648, y=w647) -> (x-y=w646:i32)
                n263 = Search 1D Array(1D array=w666, element=TRUE) -> (index of element=w664:i32)  [unwired: 1 in]
                n264 = Search 1D Array(1D array=w663, element=TRUE) -> (index of element=w660:i32)  [unwired: 1 in]
                n265 = Multiply(x=w646, y=10.0) -> (x*y=w649:dbl)
                n266 = Subtract(x=w660, y=w664) -> (x-y=w671:i32)
                n267 = for {
                  N: w649 -> [_]
                  tunnel: [w675] -> w653 mode=indexing
                  shift-right: [w675] -> _
                  shift-left: w647 -> [w676]
                  n268 = Add(x=0.1, y=w676) -> (x+y=w675:dbl)
                }
                n269 = Array Subset "Sub-positions"(array=w661, index=w664, length=w671) -> (w654:dbl[])
                n270 = Array Subset "Sub-Power"(array=w672, index=w664, length=w671) -> (w655:dbl[])
                n271 = local read "Power (mW)"() -> (w657:dbl)
                n272 = call <vilib>:"Interpolate 1D.vi"("method"=w656, "xi"=w653, "X"=w654, "Y"=w655) -> ("xi used"=w652:dbl[], "yi"=w651:dbl[])  [unwired: 5 in, 1 out]
                n273 = Build Array(w657) -> (w670:dbl[])
                n274 = call <vilib>:"Interpolate 1D.vi"("method"=w668, "xi"=w670, "X"=w651, "Y"=w652) -> ("yi"=w669:dbl[])  [unwired: 5 in, 2 out]
                n275 = Index Array(array=w669) -> (element=w659:dbl)  [unwired: 1 in]
                n276 = event shown="[1] \"Power (mW)\": Value Change" {
                  selector: _ -> [_ _]
                  dyn-events: _ -> [_ _]
                  timeout: 1 -> [_ _]
                  tunnel: w659 -> [_ w678]
                  event Timeout {
                    n277 = event-data() -> ()  [unwired: 1 in, 2 out]
                  }
                  event "Power (mW)": Value Change {
                    n278 = event-data() -> ()  [unwired: 1 in, 2 out]
                    n279 = local write "Target Position"(w678) -> ()
                  }
                }
              }
              frame #1 {
                n280 = And(x="Auto", y=w679) -> (x .and. y?=w682:bool)
                n281 = case shown="False" w682 {
                  tunnel: w683 -> [_ w685]
                  tunnel: w680 -> [w684 _]
                  frame False {
                    n282 = local write "Power (mW)"(w684) -> ()
                  }
                  frame True {
                    n283 = property on="Power (mW)" class="DigNum (strict)"("Val(Sgnl)"=w685) -> ()  [unwired: 2 in, 2 out]
                  }
                }
              }
            }
            n284 = Index Array(array=w644, index=w642) -> (element=w640:string)
            "Calibration Used" <- w640
            n285 = Build Path(base path=w641, name or relative path=w640) -> (appended path=w639:path)
            n286 = local read "Current Position"() -> (w638:sgl)
            n287 = call-poly <vilib>:"Read From Spreadsheet File.vi"("delimiter (\\t)"="," ("delimiter (\\t)"), "format (%.3f)"="%.6f", "file path (dialog if empty)"=w639) -> ("all rows"=w637:dbl[][])  [unwired: 4 in, 4 out]
            n288 = Build Array(w638) -> (w629:sgl[])
            n289 = Index Array "Power"(array=w637, index (row)=1 ("disabled index (col)")) -> (element=w628:dbl[])  [unwired: 1 in]
            n290 = Index Array "Position"(array=w637, index (row)=0 ("disabled index (col)")) -> (element=w627:dbl[])  [unwired: 1 in]
            n291 = Bundle("all rows"=w627, "all rows"=w628) -> (→"Curve":cluster{"all rows":dbl[], "all rows":dbl[]})  [unwired: 1 in]
            n292 = call <vilib>:"Interpolate 1D.vi"("method"=w632, "xi"=w629, "X"=w627, "Y"=w628) -> ("yi"=w631:dbl[])  [unwired: 5 in, 2 out]
            n293 = Index Array(array=w631) -> (element=w623:dbl)  [unwired: 1 in]
          }
        }
      }
    }
    n294 = Wait (ms)(milliseconds to wait=u32 50) -> ()  [unwired: 1 out]
  }
  n295 = call <vilib>:"DAQmx Stop Task.vi"("task/channels in"=w19, "error in"=w18) -> ()  [unwired: 12 in, 2 out]
  n296 = invoke class="MG17Motor" method="StopCtrl"(reference=w45, error in=w46) -> (error out=w44:errorcluster)  [unwired: 1 in, 2 out]
  n297 = invoke class="MG17Motor" method="StopCtrl"(reference=w25, error in=w24) -> (error out=w26:errorcluster)  [unwired: 1 in, 2 out]
  n298 = call <vilib>:"Clear Errors.vi"("error in (no error)"=w44) -> ()  [unwired: 6 in, 1 out]
  n299 = call <vilib>:"Clear Errors.vi"("error in (no error)"=w26) -> ()  [unwired: 6 in, 1 out]
  "SavePath" <- "Path"
